vi "swerve_open.vi"(8 "error in (no error)":errorcluster) -> (0 "error out":errorcluster)   [LabVIEW 2020]
uses:
  <vilib>/Rock Robotics/WPI/ThirdParty/Phoenix-LabVIEW/Pigeon IMU/CTRE_PigeonIMU_Open_CAN.vi
  Robot Global Data.vi
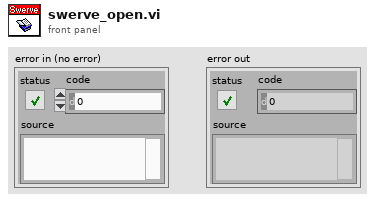
[diagram p1: front panel]
types:
  T1 = typedef "robot.ctl" = enum16{"Hyperion", "Theia"}
  T2 = typedef "CTRE_PigeonIMU_DeviceRef.ctl" = cluster{"DeviceStatus":errorcluster, "Device Number":u8, "Type":T3, "Device ID":u32, "Handle":u64, "UsageFrame":u32, "Library Path":path}
  T3 = typedef "CTRE_PigeonIMU_ConnectionType.ctl" = u32
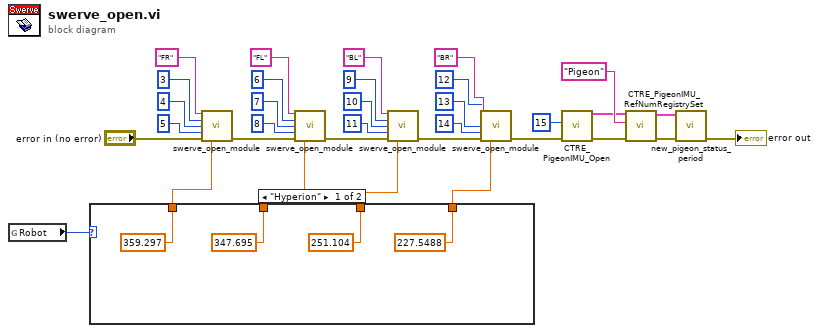
[diagram p0: block diagram]
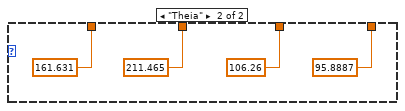
[diagram p2: hidden frame]
diagram:
  n1 = global read "Robot Global Data.vi" "Robot"() -> (w4:T1)
  n2 = case shown="\"Hyperion\"" w4 {
    tunnel: [359.297 ("Encoder Offset (Deg)") 161.631 ("Encoder Offset (Deg)")] -> w30
    tunnel: [347.695 ("Encoder Offset (Deg)") 211.465 ("Encoder Offset (Deg)")] -> w31
    tunnel: [251.104 ("Encoder Offset (Deg)") 106.26 ("Encoder Offset (Deg)")] -> w32
    tunnel: [227.5488 ("Encoder Offset (Deg)") 95.8887 ("Encoder Offset (Deg)")] -> w33
    frame "Hyperion" {
    }
    frame "Theia" {
    }
  }
  n3 = call "swerve_open_module.vi"("Module Suffix"="FR", "Drive CAN ID"=u8 3, "Azimuth CAN ID"=u8 4 ("Drive CAN ID"), "Encoder CAN ID"=u8 5 ("Drive CAN ID"), "error in"="error in (no error)", "Encoder Offset (Deg)"=w30) -> ("error out"=w17:errorcluster)  [unwired: 9 in]
  n4 = call "swerve_open_module.vi"("Module Suffix"="FL", "Drive CAN ID"=u8 6, "Azimuth CAN ID"=u8 7 ("Drive CAN ID"), "Encoder CAN ID"=u8 8 ("Drive CAN ID"), "error in"=w17, "Encoder Offset (Deg)"=w31) -> ("error out"=w22:errorcluster)  [unwired: 9 in]
  n5 = call "swerve_open_module.vi"("Module Suffix"="BL", "Drive CAN ID"=u8 9, "Azimuth CAN ID"=u8 10 ("Drive CAN ID"), "Encoder CAN ID"=u8 11 ("Drive CAN ID"), "error in"=w22, "Encoder Offset (Deg)"=w32) -> ("error out"=w27:errorcluster)  [unwired: 9 in]
  n6 = call "swerve_open_module.vi"("Module Suffix"="BR", "Drive CAN ID"=u8 12, "Azimuth CAN ID"=u8 13 ("Drive CAN ID"), "Encoder CAN ID"=u8 14 ("Drive CAN ID"), "error in"=w27, "Encoder Offset (Deg)"=w33) -> ("error out"=w28:errorcluster)  [unwired: 9 in]
  n7 = call-poly <vilib>:"CTRE_PigeonIMU_Open.vi"("error in"=w28, "Device Number"=u8 15) -> ("error out"=w7:errorcluster, "PigeonIMUDevRef"=w8:T2)  [unwired: 8 in]
  n8 = call <vilib>:"CTRE_PigeonIMU_RefNumRegistrySet.vi"("error in (no error)"=w7, "refnum name"="Pigeon", "PigeonIMUDevRef"=w8) -> ("error out"=w2:errorcluster, "PigeonIMUDevRef"=w3:T2)  [unwired: 7 in]
  n9 = call "new_pigeon_status_period.vi"("error in (no error)"=w2, "PigeonIMUDevRef In"=w3) -> ("error out"=→"error out":errorcluster)  [unwired: 8 in, 1 out]
